vi "Step`s VIs Global.vi"() -> ()   [LabVIEW 2017]
panel:
  in  "ScanBoxA.RespondSN":refnum<notifier>
  in  "ScanBoxA.RequestSN":refnum<user-event>
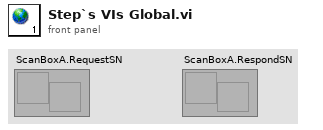
[diagram p1: front panel]
diagram:
